vi "Write body.vi"(8 "error in (no error)":errorcluster, 10 "body":string, 11 "httpRequest in":refnum<class "httpResponse.lvclass">) -> (0 "error out":errorcluster, 3 "httpRequest out":refnum<class "httpResponse.lvclass">)   [LabVIEW 2020, in "httpClient.lvlib" / "httpResponse.lvclass"]
uses:
  httpResponse.lvclass
  httpResponse.lvclass/httpResponse.ctl
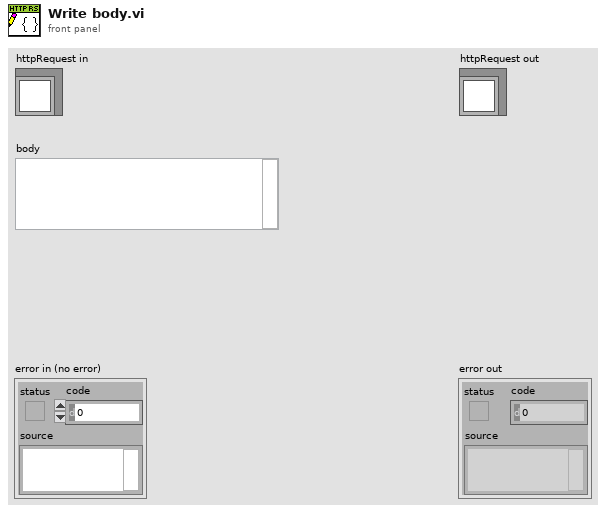
[diagram p1: front panel]
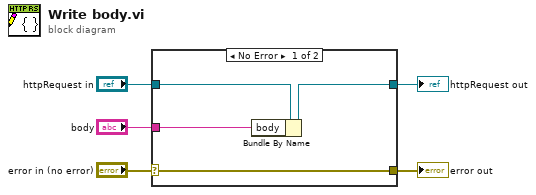
[diagram p0: block diagram]
diagram:
  n1 = case shown="No Error" "error in (no error)" {
    selector: "error in (no error)" -> [w9 w10]
    tunnel: [w9 w10] -> w4
    tunnel: [w6 w11] -> w2
    tunnel: "httpRequest in" -> [w8 w11]
    tunnel: "body" -> [w7 _]
    frame No Error {
      n2 = Bundle By Name(cluster=w8, "body"=w7) -> (w6:refnum<class "httpResponse.lvclass">)
    }
    frame Error {
    }
  }
  "error out" <- w4
  "httpRequest out" <- w2
